vi "MHR Modified Humidity Ratio Revised (Kg to Kg).vi"(1 "Gas Presure":dbl[unit]=80000.0 min=80000.0 max=120000.0, 2 "Tceg":dbl[unit], 3 "RH":dbl) -> (0 "MHR\nModified Humidity Ratio":dbl)   [LabVIEW 2018]
panel:
  out "MHR\nModified Humidity Ratio":dbl(knob) scale=0.0..1.5
  out "Temprature Of Input Air\nKelvin Degree":dbl[unit](slide) scale=273.0..373.0
  out "Tk":dbl[unit]
  out "Temprature Of Input Air\nCentigrade Degree":dbl[unit](slide) scale=0.0..100.0
  out "Humidity of Input Air":dbl(knob) scale=0.0..100.0
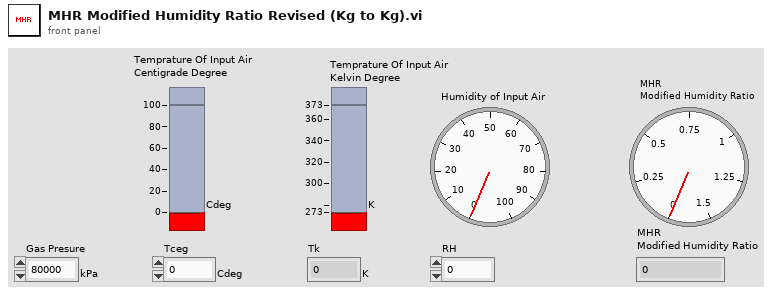
[diagram p1: front panel]
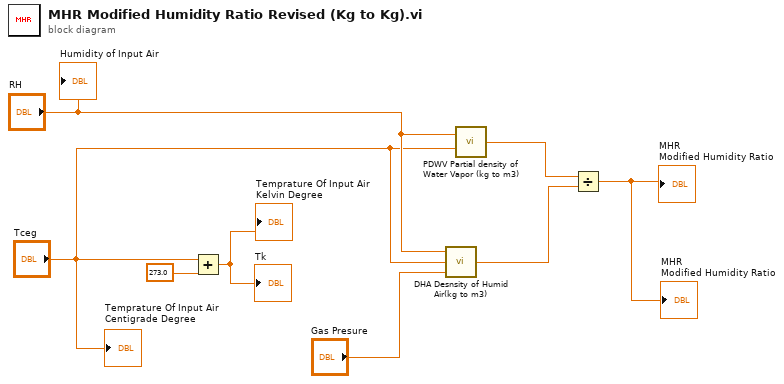
[diagram p0: block diagram]
diagram:
  n1 = Add(x="Tceg", y=dbl[unit] 273.0) -> (x+y=→"Tk" →"Temprature Of Input Air\nKelvin Degree":dbl[unit])
  n2 = call "DHA Desnsity of Humid Air(kg to m3).vi"("Total Pressure of Humid Air"="Gas Presure", "Tceg"="Tceg", "RH"="RH") -> ("DHA"=w2:dbl[unit])
  n3 = call "PDWV Partial density of Water Vapor (kg to m3).vi"("Tceg"="Tceg", "RH"="RH") -> ("PDWV"=w5:dbl[unit])
  n4 = Divide(x=w5, y=w2) -> (x/y=→"MHR\nModified Humidity Ratio" →"MHR\nModified Humidity Ratio":dbl)
  "Humidity of Input Air" <- "RH"
  "Temprature Of Input Air\nCentigrade Degree" <- "Tceg"
